vi "VisionPnPPose.vi"(5 "Turret Delta Y":dbl, 7 "Turret Delta X":dbl, 8 "Previous Y Estimate (in)":dbl, 9 "LimeLight Raw X (in)":dbl, 10 "LimeLight Raw Z (in)":dbl, 11 "Previous X Estimate (in)":dbl) -> (1 "deltaY (in)":dbl, 2 "deltaX (in)":dbl)   [LabVIEW 2019]
doc: "This VI converts the raw LimeLight pipeline values into the global field coordinate system."
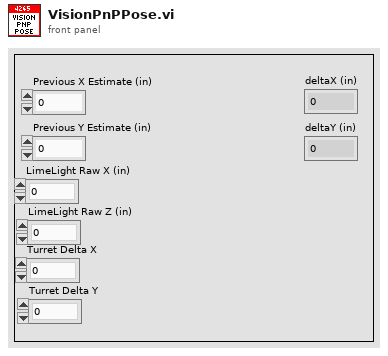
[diagram p1: front panel]
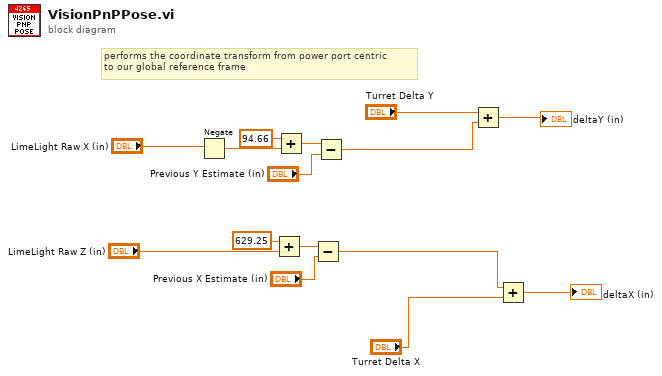
[diagram p0: block diagram]
diagram:
  # "performs the coordinate transform from power port centric\nto our global reference frame"
  n1 = Negate(x="LimeLight Raw X (in)") -> (-x=w15:dbl)
  n2 = Add(x=629.25, y="LimeLight Raw Z (in)") -> (x+y=w12:dbl)
  n3 = Add(x=94.66, y=w15) -> (x+y=w14:dbl)
  n4 = Subtract(x=w12, y="Previous X Estimate (in)") -> (x-y=w5:dbl)
  n5 = Subtract(x=w14, y="Previous Y Estimate (in)") -> (x-y=w3:dbl)
  n6 = Add(x="Turret Delta Y", y=w3) -> (x+y=→"deltaY (in)":dbl)
  n7 = Add(x=w5, y="Turret Delta X") -> (x+y=→"deltaX (in)":dbl)
